vi "Access Data.vi"(8 "error in (no error)":errorcluster, 11 "Circular Buffer 1D U16 DVR Queue in":refnum<class "Circular Buffer 1D U16 DVR Queue.lvclass">) -> (0 "error out":errorcluster, 2 "Data Out":u16[](array[numeric]), 3 "Circular Buffer 1D U16 DVR Queue out":refnum<class "Circular Buffer 1D U16 DVR Queue.lvclass">)   [LabVIEW 2019, in "Circular Buffer 1D U16 DVR Queue.lvclass"]
uses:
  Circular Buffer 1D U16 DVR Queue.lvclass
  Circular Buffer 1D U16 DVR Queue.lvclass/Circular Buffer 1D U16 DVR Queue.ctl
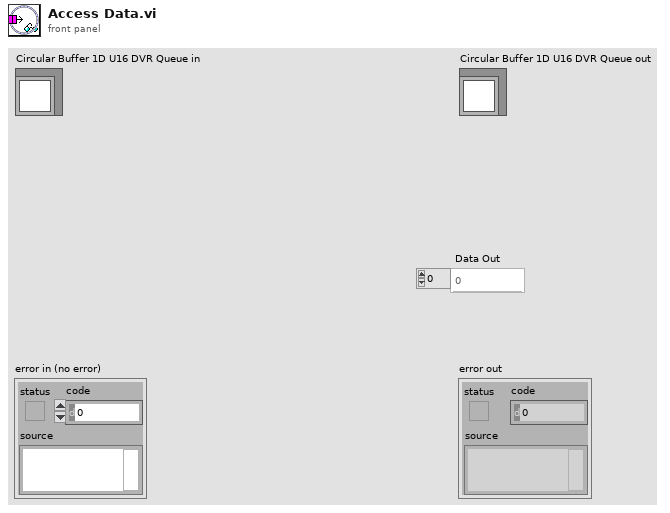
[diagram p1: front panel]
types:
  T1 = typedef "1D U16 DVR Queue.ctl" = refnum<queue>
  T2 = typedef "1D U16 DVR.ctl" = refnum<data-value>
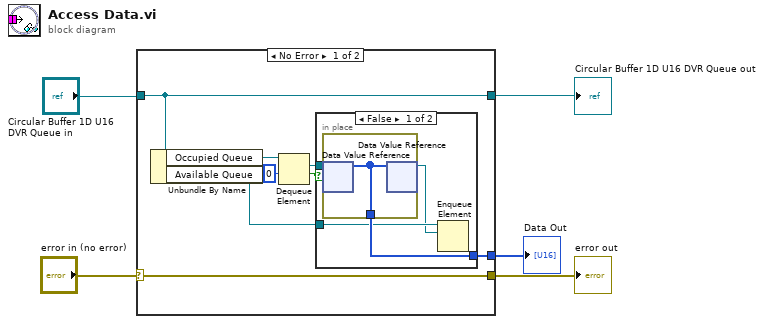
[diagram p0: block diagram]
diagram:
  n1 = case shown="No Error" "error in (no error)" {
    selector: "error in (no error)" -> [w13 w20]
    tunnel: [w13 w20] -> w2
    tunnel: [w12 w19] -> w4
    tunnel: "Circular Buffer 1D U16 DVR Queue in" -> [w12 w19]
    tunnel: [w9 _] -> w1
    frame No Error {
      n2 = Unbundle By Name(w12) -> ("Occupied Queue"=w11:T1, "Available Queue"=w8:T1)
      n3 = Dequeue Element(queue=w11, timeout in ms (-1)=0) -> (element=w10:T2, timed out?=w6:bool)  [unwired: 1 in, 2 out]
      n4 = case shown="False" w6 {
        tunnel: w10 -> [w17 _]
        tunnel: [w16 _] -> w9
        tunnel: w8 -> [w15 _]
        frame False {
          n5 = in-place {
            in-place-border: [w18] -> w16
            n6 = in-place-dvr #1(w17) -> (w18:u16[])  [unwired: 1 out]
            n7 = in-place-dvr #1(w18) -> (w14:T2)  [unwired: 1 out]
          }
          n8 = Enqueue Element(queue=w15, element=w14) -> ()  [unwired: 2 in, 3 out]
        }
        frame True {
        }
      }
    }
    frame Error {
    }
  }
  "error out" <- w2
  "Circular Buffer 1D U16 DVR Queue out" <- w4
  "Data Out" <- w1
